vi "Cross_corr.vi"(8 "m":i32=3, 9 "P":i32=9, 10 "input B":dbl[](array[numeric])=[1.0, 3.0, 5.0, 6.0, 1.0, 9.0, 0.0, 7.0, 4.0, 3.0, 9.0, 6.0, 1.0, 0.0, 0.0, 3.0, 8.0, 9.0, 2.0, 4.0, 5.0, 5.0, 1.0, 2.0, 0.0, 2.0, 3.0, 2.0, 1.0, 1.0, 0.0, 9.0, 8.0, 7.0, 4.0, 1.0, 1.0, 8.0, 9.0], 11 "input A":dbl[](array[numeric])=[1.0, 3.0, 5.0, 6.0, 1.0, 9.0, 0.0, 7.0, 4.0, 3.0, 9.0, 6.0, 1.0, 0.0, 0.0, 3.0, 8.0, 9.0, 2.0, 4.0, 5.0, 5.0, 1.0, 2.0, 0.0, 2.0, 3.0, 2.0, 1.0, 1.0, 0.0, 9.0, 8.0, 7.0, 4.0, 1.0, 1.0, 8.0, 9.0]) -> (0 "Sn A":dbl[](array[numeric]), 3 "Acc":dbl[](array[numeric]) format="%#_10g", 4 "Sn B":dbl[](array[numeric]))   [LabVIEW 2015]
panel:
  out "size(s)":i32
  out "ceil(x): smallest int >= x":dbl
  out "shift register":dbl[](array[numeric])
  out "Numeric":i32
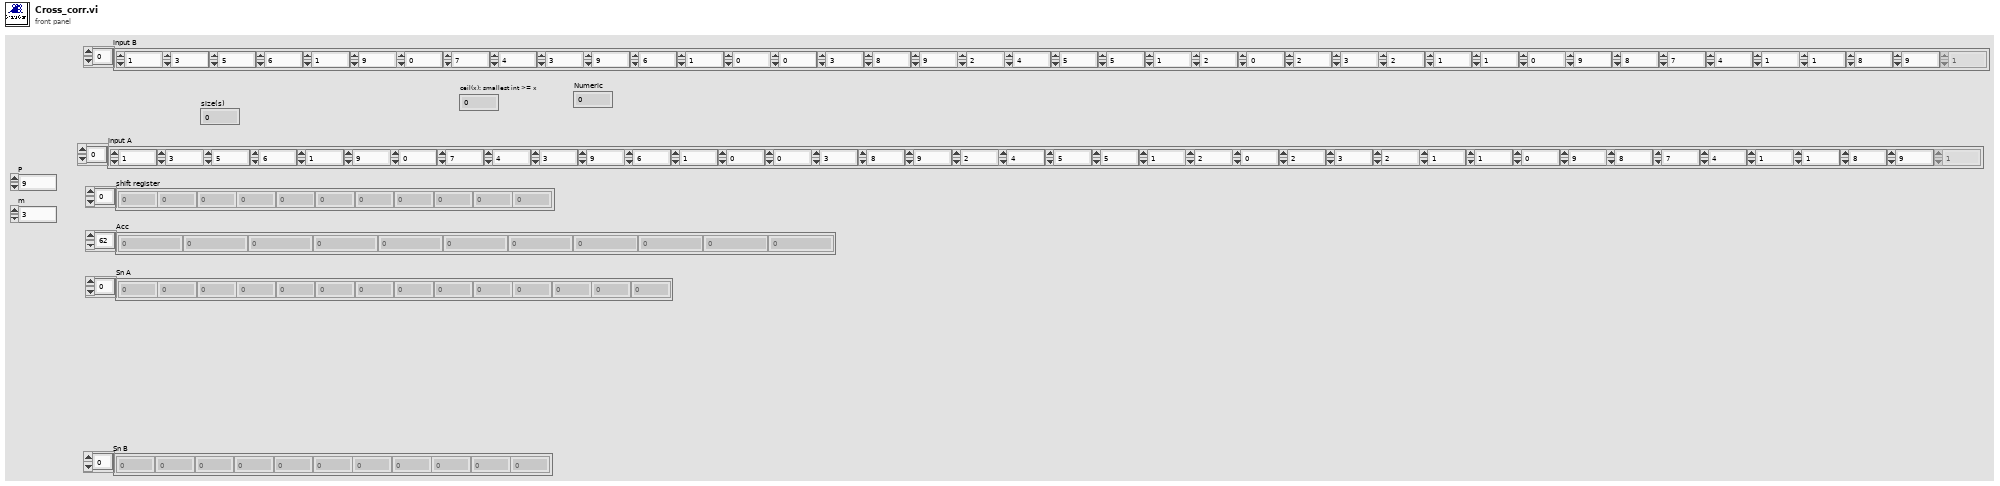
[diagram p1: front panel]
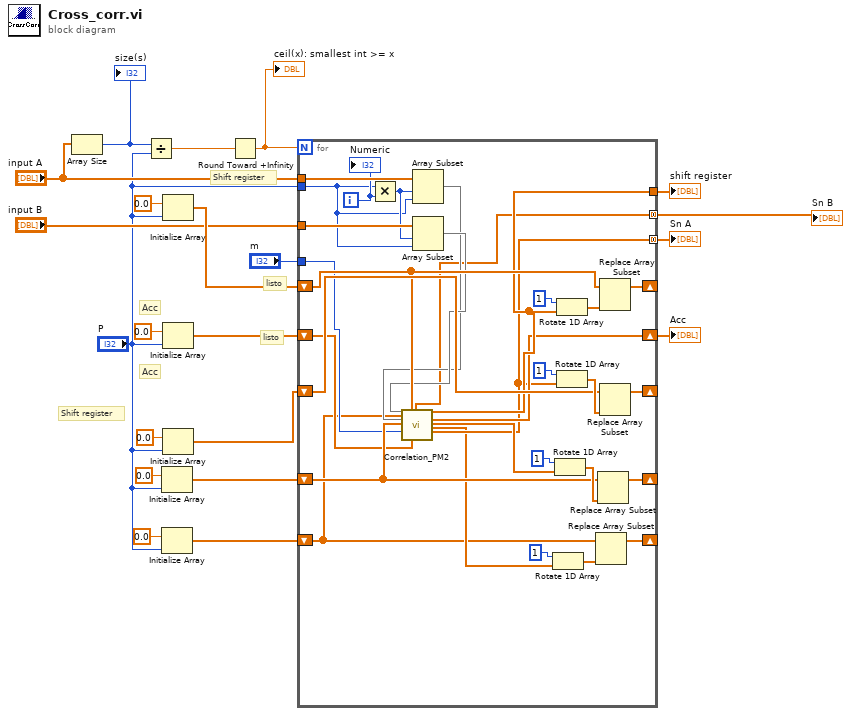
[diagram p0: block diagram]
diagram:
  # "listo"
  # "listo"
  # "Shift register"
  # "Acc"
  # "Acc"
  # "Shift register"
  n1 = Array Size(array="input A") -> (size(s)=w20:i32)
  "size(s)" <- w20
  n2 = Divide(x=w20, y="P") -> (x/y=w19:dbl)
  n3 = Initialize Array(0.0 ("dimension size"), "P") -> (w6:dbl[])
  n4 = Initialize Array(0.0 ("dimension size"), "P") -> (w2:dbl[])
  n5 = Initialize Array(0.0 ("dimension size"), "P") -> (w9:dbl[])
  n6 = Initialize Array(0.0 ("dimension size"), "P") -> (w8:dbl[])
  n7 = Initialize Array(0.0 ("dimension size"), "P") -> (w7:dbl[])
  n8 = Round Toward +Infinity(x=w19) -> (ceil(x): smallest int >= x=w18:dbl)
  "ceil(x): smallest int >= x" <- w18
  n9 = for {
    N: w18 -> [_]
    tunnel: "P" -> [w38]
    tunnel: "m" -> [w33]
    shift-right: [w50] -> _
    shift-left: w9 -> [w37]
    shift-right: [w29] -> w13
    shift-left: w8 -> [w32]
    tunnel: [w31] -> w17
    tunnel: "input A" -> [w49]
    tunnel: [w27] -> w12 mode=concatenating
    shift-right: [w46] -> _
    shift-left: w7 -> [w45]
    shift-right: [w42] -> _
    shift-left: w6 -> [w34]
    tunnel: "input B" -> [w40]
    tunnel: [w30] -> w4 mode=concatenating
    shift-right: [w22] -> _
    shift-left: w2 -> [w23]
    i -> [w41]
    n10 = Multiply(x=w38, y=w41) -> (x*y=w39:i32)
    n11 = Array Subset(array=w49, index=w39, length=w38) -> (w35:dbl[])
    n12 = Array Subset(array=w40, index=w39, length=w38) -> (w36:dbl[])
    n13 = call "Correlation_PM2.vi"("Input B"=w36, "shift register D"=w23, "Input A"=w35, "shift register MY"=w34, "m"=w33, "shift register in"=w37, "Acc in"=w32) -> ("MnB"=w30:dbl[], "shift register"=w31:dbl[], "Acc"=w29:dbl[], "shift register Y out"=w28:dbl[], "shift register out D"=w24:dbl[], "MnA"=w27:dbl[])  [unwired: 15 in]
    n14 = Rotate 1D Array(1:w24, 2:1 ("n")) -> (0:w25:dbl[])
    n15 = Rotate 1D Array(1:w28, 2:1 ("n")) -> (0:w43:dbl[])
    n16 = Rotate 1D Array(1:w31, 2:1 ("n")) -> (0:w51:dbl[])
    n17 = Rotate 1D Array(1:w27, 2:1 ("n")) -> (0:w47:dbl[])
    n18 = Replace Array Subset(array=w23, new element=w25) -> (w22:dbl[])  [unwired: 1 in]
    n19 = Replace Array Subset(array=w34, new element=w43) -> (w42:dbl[])  [unwired: 1 in]
    n20 = Replace Array Subset(array=w37, new element=w51) -> (w50:dbl[])  [unwired: 1 in]
    n21 = Replace Array Subset(array=w45, new element=w47) -> (w46:dbl[])  [unwired: 1 in]
    "Numeric" <- w41
  }
  "shift register" <- w17
  "Acc" <- w13
  "Sn A" <- w12
  "Sn B" <- w4
